vi "Destroy.vi"(0 "reference in":refnum<class "CondimentDecorator.lvclass">, 5 "error in (no error)":errorcluster) -> (14 "reference out":refnum<class "CondimentDecorator.lvclass">, 19 "error out":errorcluster)   [LabVIEW 2020, in "CondimentDecorator.lvclass"]
uses:
  CondimentDecorator.lvclass
  Beverage_class/Beverage.lvclass
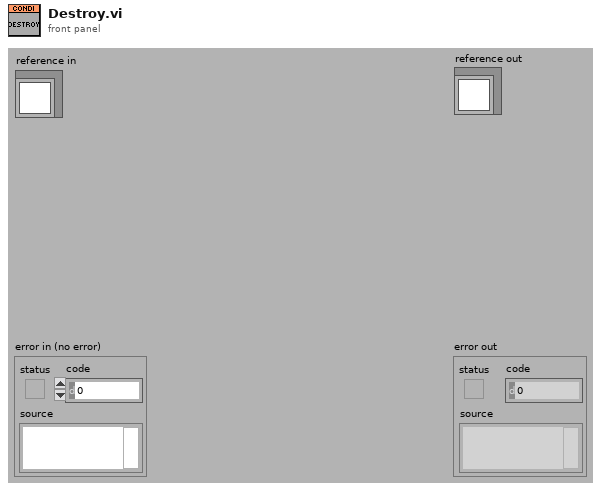
[diagram p1: front panel]
types:
  T1 = typedef "CondimentDecorator.lvclass/ObjectAttributes.ctl" = cluster{"BeverageRef":refnum<class "Beverage.lvclass">, "CondimentName":string}
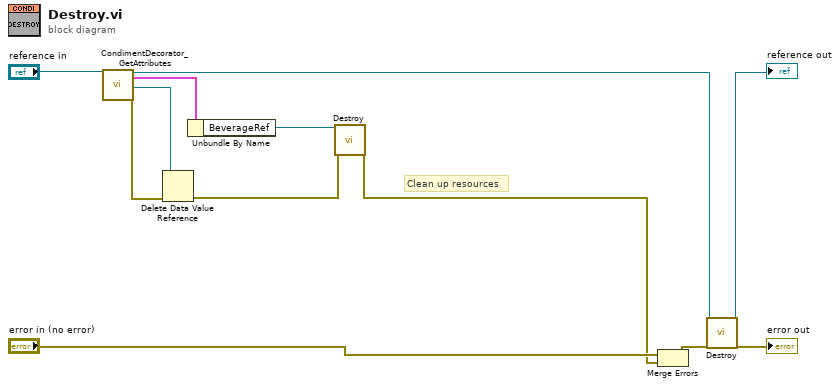
[diagram p0: block diagram]
diagram:
  # "Clean up resources"
  n1 = call "CondimentDecorator_GetAttributes.vi"("reference in"="reference in") -> ("reference out"=w6:refnum<class "CondimentDecorator.lvclass">, "Data"=w9:T1, "DataRef"=w10:refnum<data-value>, "error out"=w11:errorcluster)  [unwired: 15 in]
  n2 = Delete Data Value Reference(data value reference=w10, error in=w11) -> (error out=w2:errorcluster)  [unwired: 1 out]
  n3 = Unbundle By Name(w9) -> ("BeverageRef"=w3:refnum<class "Beverage.lvclass">)
  n4 = call-dynamic "Destroy.vi"("reference in"=w3, "error in (no error)"=w2) -> ("error out"=w1:errorcluster)  [unwired: 16 in, 1 out]
  n5 = Merge Errors("error in (no error)", w1) -> (w8:errorcluster)
  n6 = call-parent "Destroy.vi"("reference in"=w6, "error in (no error)"=w8) -> ("reference out"=→"reference out":refnum<class "CondimentDecorator.lvclass">, "error out"=→"error out":errorcluster)  [unwired: 16 in]
